vi "Configure Output Timer.vi"(5 "Duration (1 s)":i32=1, 6 "Current Level (0 A)":dbl, 7 "Voltage Level (0 V)":dbl, 8 "error in (no error)":errorcluster, 9 "Timer Number (1)":i32=1, 10 "Channel (0: 30V Channel)":T1 caption="Channel (0: +6V)" items=["30V/3A Channel", "30V/3A Channel", "5V/3A Channel"], 11 "VISA resource name":refnum<visa-resource-name>) -> (0 "error out":errorcluster, 3 "VISA resource name out":refnum<visa-resource-name>)   [LabVIEW 2020, in "RIGOL DP800 Series.lvlib"]
doc: "Configures the output timer function."
uses:
  <instrlib>/RIGOL DP800 Series/RIGOL DP800 Series.lvlib
  <instrlib>/RIGOL DP800 Series/Public/Channels.ctl
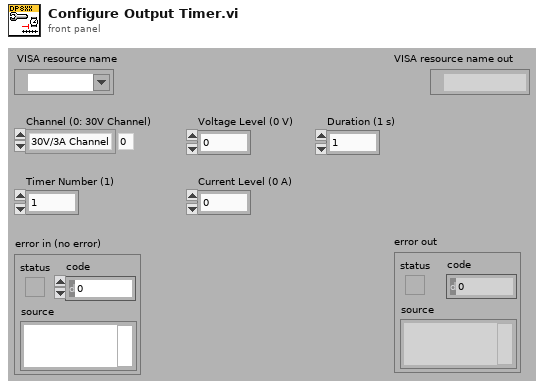
[diagram p1: front panel]
types:
  T1 = typedef "RIGOL DP800 Series.lvlib/Channels.ctl" = i32
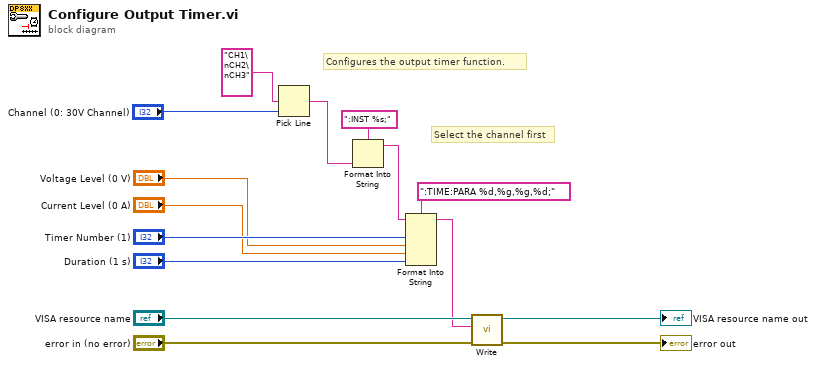
[diagram p0: block diagram]
diagram:
  # "Select the channel first"
  # "Configures the output timer function."
  n1 = Pick Line(multi-line string="CH1\nCH2\nCH3", line index="Channel (0: 30V Channel)") -> (output string=w3:string)  [unwired: 1 out]
  n2 = Format Into String(format string=":INST %s;", w3) -> (resulting string=w2:string)  [unwired: 2 in, 1 out]
  n3 = Format Into String(format string=":TIME:PARA %d,%g,%g,%d;", initial string=w2, "Timer Number (1)", "Voltage Level (0 V)", "Current Level (0 A)", "Duration (1 s)") -> (resulting string=w1:string)  [unwired: 1 in, 1 out]
  n4 = call <instrlib>:"Write.vi"("error in (no error)"="error in (no error)", "Write Buffer (\"\")"=w1, "VISA resource name"="VISA resource name") -> ("error out"=→"error out":errorcluster, "VISA resource name out"=→"VISA resource name out":refnum<visa-resource-name>)  [unwired: 7 in]
